vi "gyro -- async sweeper.vi"(11 "sweeper event pair":T4) -> ()   [LabVIEW 2018]
uses:
  gyro -- async sweeper parameters.ctl
  freq scan type.ctl
  show-win- control.ctl
  server talk-to-back pair.ctl
  server talkback message type.ctl
  server talkto message type.ctl
  publisher action.ctl
  data source action.ctl
  array - generate range.vi
  array -- sort 2D array -- Complex.vi/05c44075-957c-bc42-b6fa-2799d0bc0485.vi
  <vilib>/Array/Sort 2D Array - Pop Stack.vi
  <vilib>/Array/Sort 2D Array - Push Stack.vi
  array -- sort 2D array -- Complex.vi/05c44075-957c-bc42-b6fa-2799d0bc0485.vi/cccbd045-f7a0-8040-9e33-9155ef8dc433.vi
  array -- sort 2D array -- Complex.vi/05c44075-957c-bc42-b6fa-2799d0bc0485.vi/c298cb75-c0bc-c146-b830-07b0d605e302.vi
panel:
  in  "Tab Control":enum32{"Page 1", "Page 2"}(tab)
  in  "sweeper parameters":T1={"delay-circle(msec)"=0, "N"=300, "scan type"=enum."linear", "gamma factor"=1.5, "history length"=1}
  in  "win":T3={"cen (Hz)"=32757.83435625395, "win (Hz)"=134.34356253945762, "left (Hz)"=32690.66257498422, "right (Hz)"=32825.00613752368}
  out "progress":i32(slide) min=0 max=300 step=1 scale=0.0..300.0
  out "stopped?":bool=TRUE
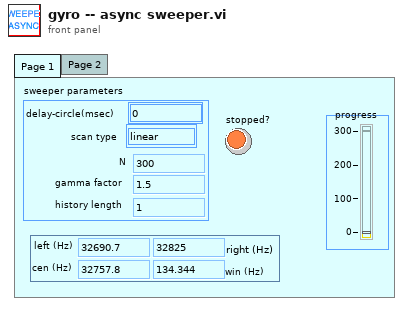
[diagram p1: front panel]
types:
  T1 = typedef "gyro -- async sweeper parameters.ctl" = cluster{"delay-circle(msec)":i64, "N":i64, "scan type":T2, "gamma factor":dbl, "history length":i64}
  T2 = typedef "freq scan type.ctl" = enum16{"linear", "arctan"}
  T3 = typedef "show-win- control.ctl" = cluster{"cen (Hz)":dbl, "win (Hz)":dbl, "left (Hz)":dbl, "right (Hz)":dbl}
  T4 = typedef "server talk-to-back pair.ctl" = cluster{"talkback event":refnum<user-event>, "talkto event":refnum<user-event>}
  T5 = typedef "publisher action.ctl" = enum16{"set", "get", "init", "check"}
  T6 = typedef "server talkback message type.ctl" = cluster{"message":enum16{"new", "void"}}
  T7 = typedef "data source action.ctl" = enum16{"set", "get", "init", "set-and-get", "init source"}
  T8 = enum16{"stop", "start", "update pars", "update request", "new", "launch", "exit", "get", "reset", "pause", "unpause"}
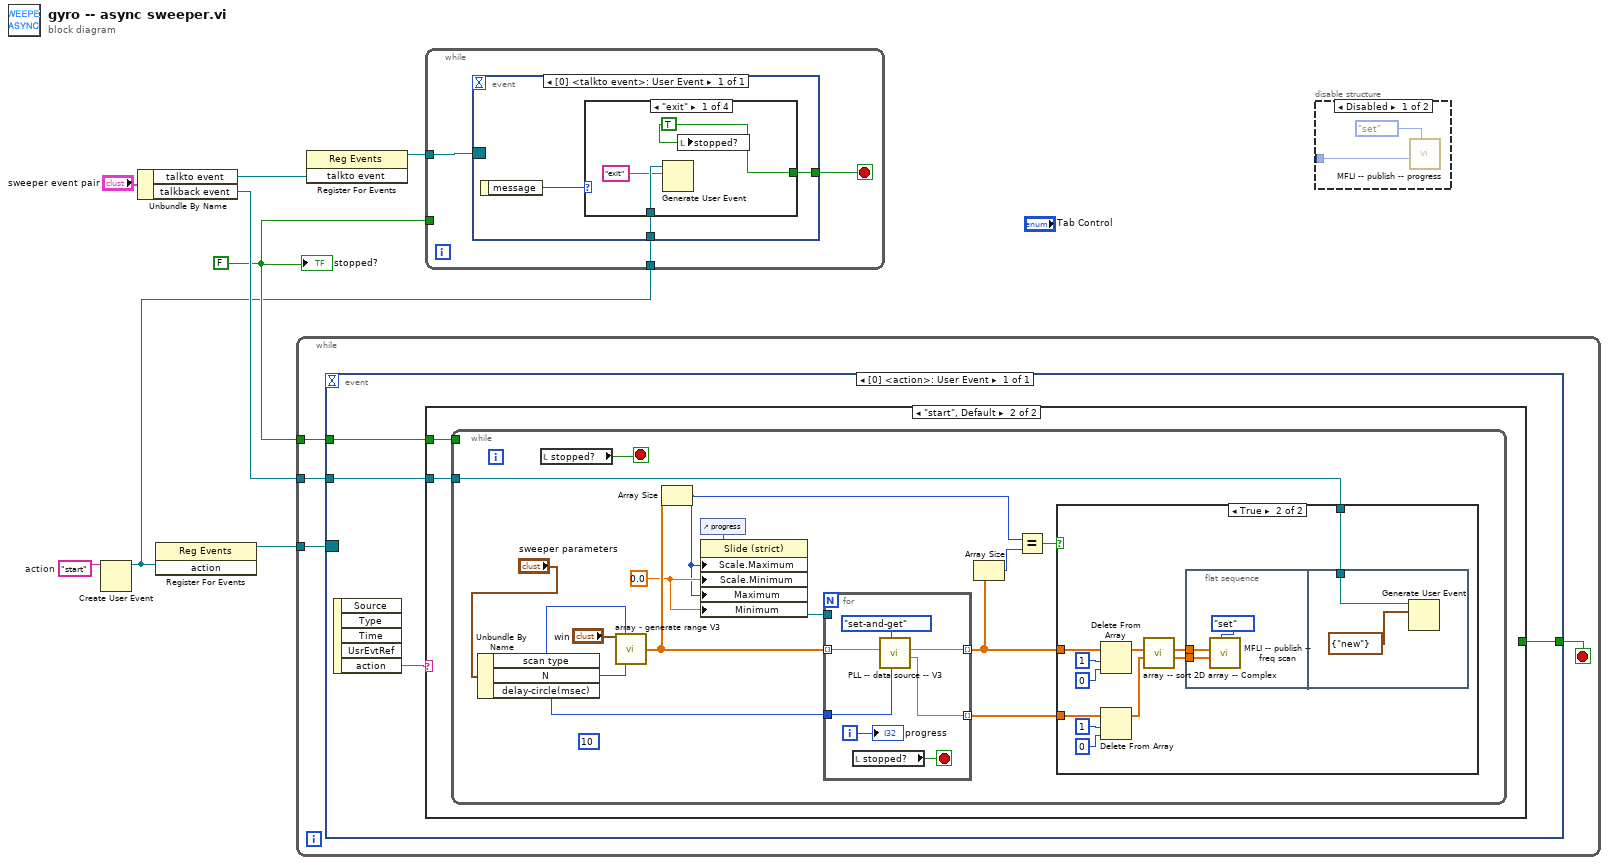
[diagram p0: block diagram]
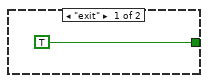
[diagram p2: hidden frame]
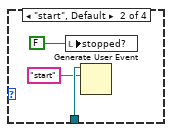
[diagram p5: hidden frame]
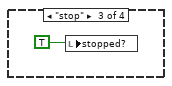
[diagram p6: hidden frame]
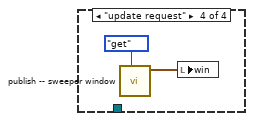
[diagram p7: hidden frame]
diagram:
  w3 = "start"  # action
  w2 = FALSE ("stop!")
  n1 = Create User Event(user event datatype=w3) -> (user event=w1:refnum<user-event>)  [unwired: 1 in, 1 out]
  n2 = Unbundle By Name("sweeper event pair") -> ("talkto event"=w6:refnum<user-event>, "talkback event"=w5:refnum<user-event>)
  n3 = register-events(w1) -> (reference out=w4:refnum<event-registration>)  [unwired: 2 in, 1 out]
  n4 = while {
    tunnel: w2 -> [w12]
    tunnel: w5 -> [w11]
    tunnel: w4 -> [w10]
    stop <- w9 stop-if-true
    n5 = event shown="[0] <action>: User Event" {
      selector: w10 -> [_]
      dyn-events: _ -> [_]
      timeout: _ -> [_]
      tunnel: w12 -> [w16]
      tunnel: w11 -> [w15]
      tunnel: [w13] -> w9
      event User Event {
        n6 = event-data() -> ("action"=w14:string)  [unwired: 1 in, 4 out]
        n7 = case shown="\"start\", Default" w14 {
          tunnel: w16 -> [_ w19]
          tunnel: w15 -> [_ w18]
          tunnel: [TRUE ("stop!") _] -> w13
          frame "exit" {
          }
          frame "start", Default {
            n8 = while {
              tunnel: w19 -> [_]
              tunnel: w18 -> [w33]
              stop <- w25 stop-if-true
              (unwired) 10 ("lower")
              w27 = 0.0 ("Scale.Range:Minimum")
              n9 = Unbundle By Name("sweeper parameters") -> ("scan type"=w32:T2, "N"=w20:i64, "delay-circle(msec)"=w31:i64)
              n10 = local read "stopped?"() -> (w25:bool)
              n11 = call "array - generate range V3.vi"("win"="win", "scan type"=w32, "N"=w20) -> ("Array"=w29:dbl[])  [unwired: 11 in, 1 out]
              n12 = Array Size(array=w29) -> (size(s)=w21:i32)
              n13 = control-ref of="progress"() -> (w30:refnum<vi>)
              n14 = property class="Slide (strict)"(reference=w30, "Scale.Maximum"=w21, "Scale.Minimum"=w27, "Maximum"=w21, "Minimum"=w27) -> (reference out=w28:refnum<vi>)  [unwired: 1 in, 1 out]
              n15 = for {
                tunnel: w29 -> [w54] mode=indexing
                tunnel: w31 -> [w56]
                tunnel: [w58] -> w35 mode=indexing
                tunnel: [w57] -> w24 mode=indexing
                tunnel: w28 -> [_]
                i -> [w53]
                stop <- w52 stop-if-true
                n16 = local read "stopped?"() -> (w52:bool)
                n17 = call "PLL -- data source -- V3.vi"("set-get delay (msec)"=w56, "data source action"=data_source_action."set-and-get", "Freq in (Hz)"=w54) -> ("z out (V)"=w58:cdb, "Freq out (Hz)"=w57:dbl)  [unwired: 6 in, 1 out]
                "progress" <- w53
              }
              n18 = Array Size(array=w24) -> (size(s)=w22:i32)
              n19 = Equal?(x=w21, y=w22) -> (x = y?=w23:bool)
              n20 = case shown="True" w23 {
                tunnel: w35 -> [_ w42]
                tunnel: w24 -> [_ w41]
                tunnel: w33 -> [_ w36]
                frame False {
                }
                frame True {
                  n21 = Delete From Array(array=w41, length=1, index=0) -> (array with subset deleted=w40:dbl[])  [unwired: 1 out]
                  n22 = Delete From Array(array=w42, length=1, index=0) -> (array with subset deleted=w39:cdb[])  [unwired: 1 out]
                  n23 = call "array -- sort 2D array -- Complex.vi"("z In"=w39, "freq IN"=w40) -> ("z out"=w37:cdb[], "freq out"=w38:dbl[])  [unwired: 8 in]
                  n24 = flat-sequence {
                    tunnel: w37 -> [w48]
                    tunnel: w38 -> [w47]
                    tunnel: w36 -> [w51]
                    frame #0 {
                      n25 = call "MFLI -- publish -- freq scan.vi"("publisher action"=publisher_action."set", "Voltage IN (V)"=w48, "Freq IN (Hz)"=w47) -> ()  [unwired: 7 in, 2 out]
                    }
                    frame #1 {
                      n26 = Generate User Event(user event=w51, event data cluster=T6 {"message"=enum."new"} ("event data")) -> ()  [unwired: 2 in, 2 out]
                    }
                  }
                }
              }
            }
          }
        }
      }
    }
  }
  n27 = register-events(w6) -> (reference out=w8:refnum<event-registration>)  [unwired: 2 in, 1 out]
  n28 = while {
    tunnel: w8 -> [w61]
    tunnel: w2 -> [_]
    tunnel: w1 -> [w59]
    stop <- w60 stop-if-true
    n29 = event shown="[0] <talkto event>: User Event" {
      selector: w61 -> [_]
      dyn-events: _ -> [_]
      timeout: _ -> [_]
      tunnel: [w64] -> w60
      tunnel: w59 -> [w62]
      event User Event {
        n30 = event-data() -> ("message"=w63:T8)  [unwired: 1 in]
        n31 = case shown="\"exit\"" w63 {
          tunnel: [w67 _ _ _] -> w64
          tunnel: w62 -> [w66 w69 _ _]
          frame "exit" {
            w67 = TRUE ("stop!")
            n32 = Generate User Event(user event=w66, event data cluster="exit" ("event data")) -> ()  [unwired: 2 in, 2 out]
            n33 = local write "stopped?"(w67) -> ()
          }
          frame "start", Default {
            n34 = local write "stopped?"(FALSE ("stop!")) -> ()
            n35 = Generate User Event(user event=w69, event data cluster="start" ("event data")) -> ()  [unwired: 2 in, 2 out]
          }
          frame "stop" {
            n36 = local write "stopped?"(TRUE ("stop!")) -> ()
          }
          frame "update request" {
            n37 = call "publish -- sweeper window.vi"("publisher action"=publisher_action."get") -> ("win OUT"=w72:T3)  [unwired: 10 in]
            n38 = local write "win"(w72) -> ()
          }
        }
      }
    }
  }
  n39 = disable-structure shown="Disabled" {
    disable-tunnel: _ -> [w74 _]
    frame Disabled {
      n40 = call "MFLI -- publish -- progress.vi"("publisher action"=publisher_action."set", "num"=w74) -> ()  [unwired: 9 in, 1 out]
    }
    frame Enabled {
    }
  }
  "stopped?" <- w2
